vi "Generate BitfilePath.vi"() -> (0 "Bitfile path":path)   [LabVIEW 2018, in "FPGA Addon DMA Channels Basic System Tests.lvclass"]
uses:
  FPGA Addon DMA Channels Basic System Tests.lvclass
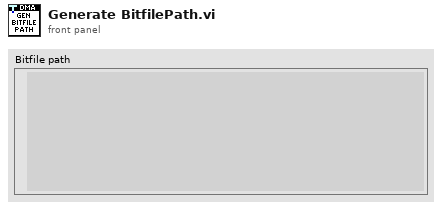
[diagram p1: front panel]
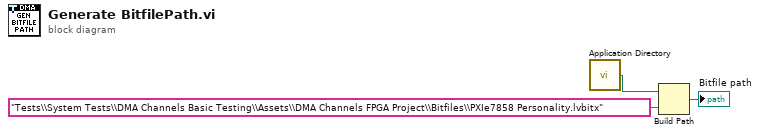
[diagram p0: block diagram]
diagram:
  n1 = call <vilib>:"Application Directory.vi"() -> ("Application Directory"=w3:path)
  n2 = Build Path(base path=w3, name or relative path="Tests\\System Tests\\DMA Channels Basic Testing\\Assets\\DMA Channels FPGA Project\\Bitfiles\\PXIe7858 Personality.lvbitx") -> (appended path=→"Bitfile path":path)
